vi "Get Path To User Service Template Library.vi"() -> (0 "appended path":path)   [LabVIEW 2019, in "gRPC Template Creation Utility.lvlib"]
uses:
  gRPC Template Creation Utility.lvlib
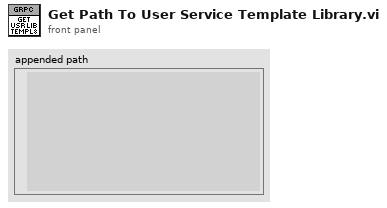
[diagram p1: front panel]
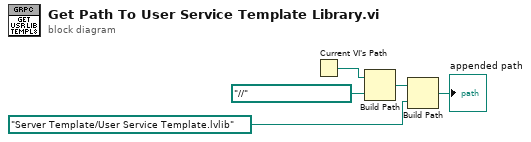
[diagram p0: block diagram]
diagram:
  n1 = Current VI's Path() -> (path=w5:path)
  n2 = Build Path(base path=w5, name or relative path=path "../../..") -> (appended path=w4:path)
  n3 = Build Path(base path=w4, name or relative path=path "Server Template/User Service Template.lvlib") -> (appended path=→"appended path":path)
